vi "Enable or Disable Buttons.vi"(8 "Error In":errorcluster, 10 "Disable?":bool=TRUE, 11 "Refnum array":refnum<vi>[](array[refnum])) -> (0 "Error Out":errorcluster, 3 "Refnum Out":refnum<vi>[](array[refnum]))   [LabVIEW 2024]
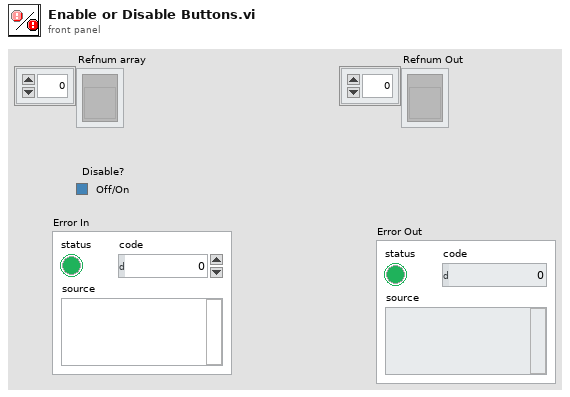
[diagram p1: front panel]
types:
  T1 = enum8{"Enabled", "Disabled", "Disabled and Grayed Out"}
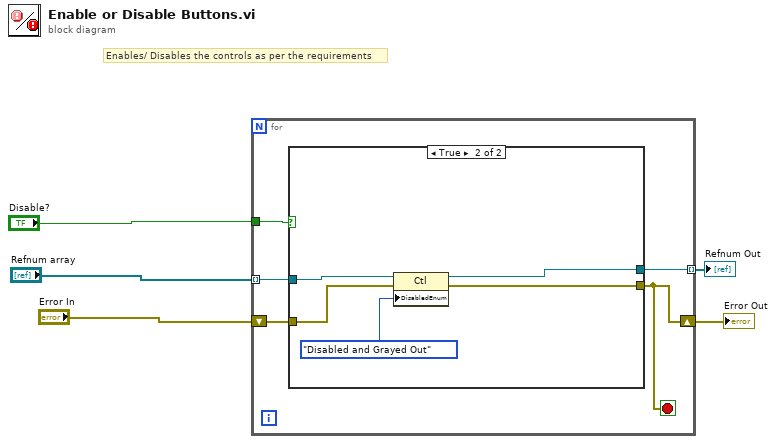
[diagram p0: block diagram]
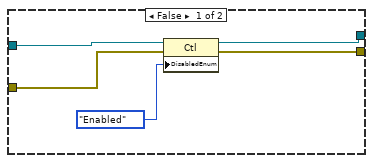
[diagram p2: hidden frame]
diagram:
  # "Enables/ Disables the controls as per the requirements"
  n1 = for {
    tunnel: "Refnum array" -> [w10] mode=indexing
    tunnel: "Disable?" -> [w8]
    shift-right: [w7] -> w2
    shift-left: "Error In" -> [w9]
    tunnel: [w6] -> w1 mode=indexing
    stop <- w7 stop-if-true
    n2 = case shown="True" w8 {
      tunnel: w10 -> [w14 w20]
      tunnel: w9 -> [w13 w19]
      tunnel: [w12 w17] -> w7
      tunnel: [w11 w16] -> w6
      frame False {
        n3 = property class="Ctl"(reference=w14, error in=w13, "DisabledEnum"=T1."Enabled" ("Disabled")) -> (reference out=w11:refnum<vi>, error out=w12:errorcluster)
      }
      frame True {
        n4 = property class="Ctl"(reference=w20, error in=w19, "DisabledEnum"=T1."Disabled and Grayed Out" ("Disabled")) -> (reference out=w16:refnum<vi>, error out=w17:errorcluster)
      }
    }
  }
  "Error Out" <- w2
  "Refnum Out" <- w1
